vi "run path.vi"(8 "error in (no error)":errorcluster, 10 "Path Number":i32, 11 "Stepper in":refnum<class "Stepper.lvclass">) -> (0 "error out":errorcluster, 3 "Stepper out":refnum<class "Stepper.lvclass">)   [LabVIEW 2025, in "Motor.lvlib" / "Stepper.lvclass"]
uses:
  Stepper.lvclass
  Stepper.lvclass/Stepper.ctl
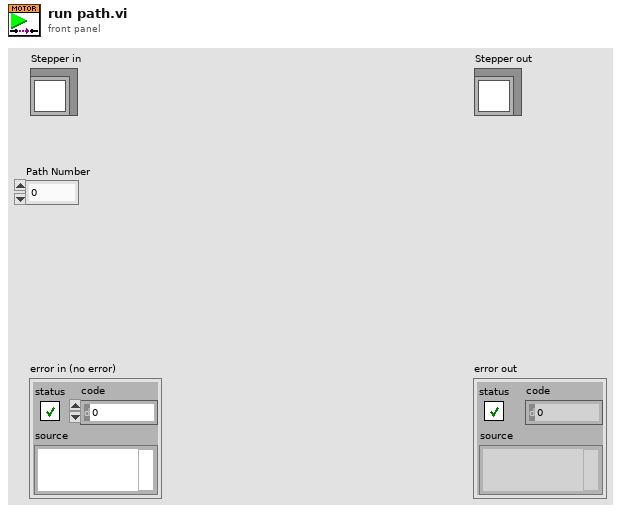
[diagram p1: front panel]
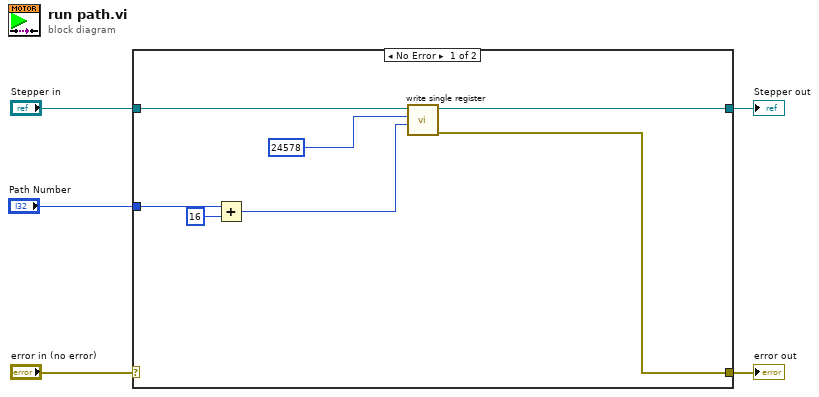
[diagram p0: block diagram]
diagram:
  n1 = case shown="No Error" "error in (no error)" {
    selector: "error in (no error)" -> [_ w14]
    tunnel: [w10 w14] -> w4
    tunnel: [w11 w13] -> w2
    tunnel: "Stepper in" -> [w12 w13]
    tunnel: "Path Number" -> [w8 _]
    frame No Error {
      n2 = Add(x=w8, y=16) -> (x+y=w6:i32)
      n3 = call-dynamic "write single register.vi"("register to write"=w6, "address"=u16 24578, "Stepper in"=w12) -> ("error out"=w10:errorcluster, "Stepper out"=w11:refnum<class "Stepper.lvclass">)  [unwired: 7 in]
    }
    frame Error {
    }
  }
  "error out" <- w4
  "Stepper out" <- w2
